vi "auto phase.vi"(8 "error in (no error)":errorcluster, 11 "VISA resource name":refnum<visa-resource-name>) -> (0 "error out":errorcluster, 2 "return phase":string, 3 "VISA resource name out":refnum<visa-resource-name>)   [LabVIEW 2014]
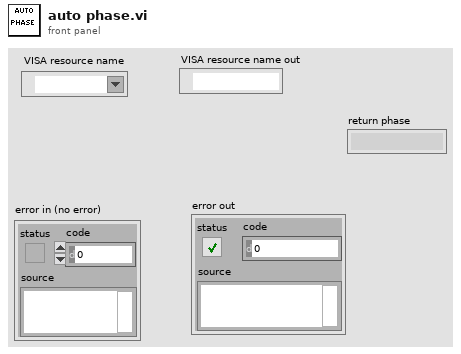
[diagram p1: front panel]
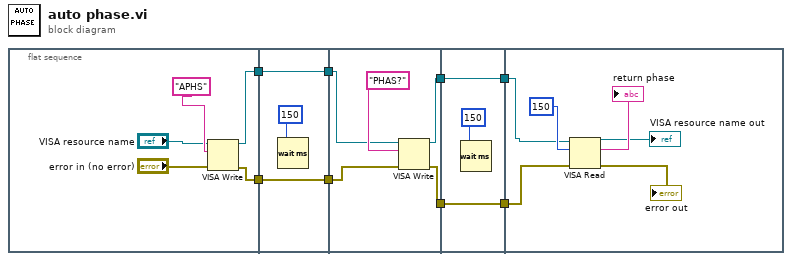
[diagram p0: block diagram]
diagram:
  n1 = flat-sequence {
    tunnel: [w10] -> w7
    tunnel: [w9] -> w5
    tunnel: [w15] -> w8
    tunnel: w7 -> [w15]
    tunnel: [w14] -> w6
    tunnel: w5 -> [w14]
    tunnel: w8 -> [w20]
    tunnel: w6 -> [w19]
    tunnel: [w18] -> w3
    tunnel: [w17] -> w1
    tunnel: [w23] -> w4
    tunnel: w3 -> [w23]
    tunnel: [w22] -> w2
    tunnel: w1 -> [w22]
    tunnel: w4 -> [w26]
    tunnel: w2 -> [w25]
    frame #0 {
      n2 = VISA Write(VISA resource name="VISA resource name", write buffer="APHS" ("format string"), error in (no error)="error in (no error)") -> (VISA resource name out=w10:refnum<visa-resource-name>, error out=w9:errorcluster)  [unwired: 1 out]
    }
    frame #1 {
      n3 = Wait (ms)(milliseconds to wait=u32 150) -> ()  [unwired: 1 out]
    }
    frame #2 {
      n4 = VISA Write(VISA resource name=w20, write buffer="PHAS?" ("format string"), error in (no error)=w19) -> (VISA resource name out=w18:refnum<visa-resource-name>, error out=w17:errorcluster)  [unwired: 1 out]
    }
    frame #3 {
      n5 = Wait (ms)(milliseconds to wait=u32 150) -> ()  [unwired: 1 out]
    }
    frame #4 {
      n6 = VISA Read(VISA resource name=w26, byte count=u32 150, error in (no error)=w25) -> (VISA resource name out=→"VISA resource name out":refnum<visa-resource-name>, read buffer=→"return phase":string, error out=→"error out":errorcluster)  [unwired: 1 out]
    }
  }
